vi "Complex LU Factor.vi"(0 "A":T1) -> (1 "LU Info":cluster{"LU":cdb[][], "Pivot":i32[]} {"LU" format="%.3f"}, 2 "sign":i32, 3 "error":i32)   [LabVIEW 2018, in "NI_AALBase.lvlib"]
doc: "Performs the cross multiplication of two input matrices. If A represents the first input matrix, B the second input, and C the resulting output matrix, the elements of C are determined according to the following equation\n\n C[i,j] = Sum{ A[i,l] B[l,j] } for l = 0, 1, 2, ...k-1\n\n where\n k is the number of columns in A and the number of rows in\n B\n j ranges from 0 to (number of columns in B - 1)\n i ranges from 0 to (number of rows in A - 1)."
uses:
  NI_AALBase.lvlib
  ComplexMatrix.ctl
  <resource>/lvanlys.dll
  NI_Matrix.lvlib
panel:
  # "Complex LU Factor"
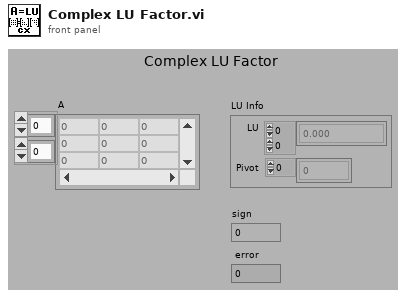
[diagram p1: front panel]
types:
  T1 = typedef "NI_Matrix.lvlib/ComplexMatrix.ctl" = cdb[][]
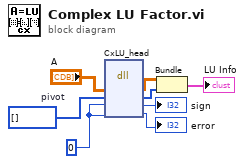
[diagram p0: block diagram]
diagram:
  w6 = i32[] []  # pivot
  w3 = 0
  n1 = dll-call lib="C:/Program Files (x86)/National Instruments/LabVIEW 2018/resource/lvanlys.*" fn="CxLU_head"("A"="A", "pivot"=w6, w3, w3) -> ("A"=w7:T1, "pivot"=w5:i32[], →"sign":i32, →"error":i32)  [unwired: 4 in, 2 out]
  n2 = Bundle("A"=w7, "pivot"=w5) -> (→"LU Info":cluster{"A":T1, "pivot":i32[]})  [unwired: 1 in]
